vi "XNET Create Timing Source (FlexRay Cycle).vi"(0 "session in":refnum<k21>, 1 "timing source name":string, 7 "macrotick offset":u32, 11 "error in (no error)":errorcluster) -> (4 "session out":refnum<k21>, 6 "timing source out":string, 15 "error out":errorcluster)   [LabVIEW 2018]
doc: "Creates a timing source for a Timed Loop on LabVIEW Real-Time.\n\nThe timing source is based on the FlexRay communication cycle. The timing source sends a tick to the Timed Loop at a specific offset in time within the FlexRay cycle. The offset within the cycle is specified in FlexRay macroticks."
uses:
  nixlvapi.dll
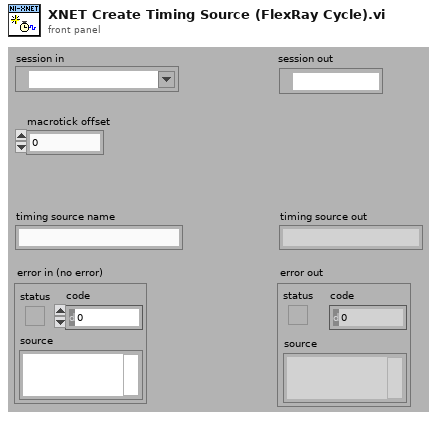
[diagram p1: front panel]
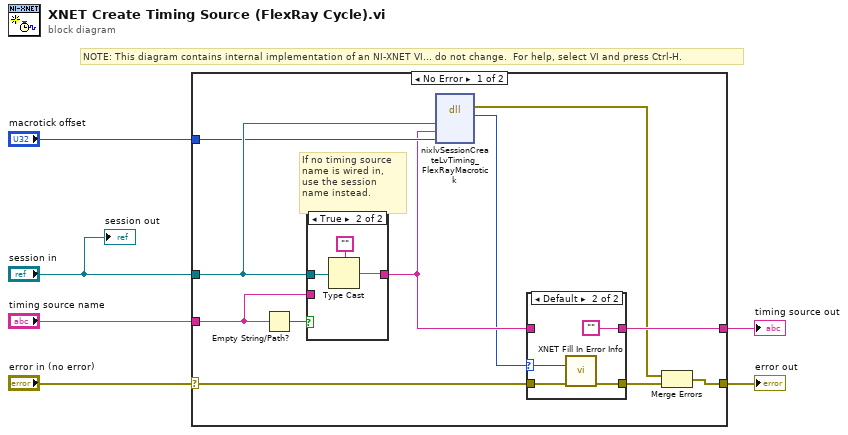
[diagram p0: block diagram]
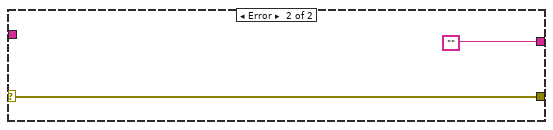
[diagram p4: hidden frame]
diagram:
  # "NOTE: This diagram contains internal implementation of an NI-XNET VI... do not change.  For help, select VI and press Ctrl-H."
  n1 = case shown="No Error" "error in (no error)" {
    selector: "error in (no error)" -> [w17 w29]
    tunnel: [w8 w29] -> w5
    tunnel: "timing source name" -> [w14 _]
    tunnel: "session in" -> [w12 _]
    tunnel: "macrotick offset" -> [w11 _]
    tunnel: [w13 ""] -> w1
    frame No Error {
      # "If no timing source \nname is wired in,\nuse the session \nname instead."
      # "NOTE: This diagram contains internal implementation of an NI-XNET VI... do not change.  For help, select VI and press Ctrl-H."
      n2 = Empty String/Path?(string/path=w14) -> (empty?=w15:bool)
      n3 = case shown="True" w15 {
        tunnel: w12 -> [_ w21]
        tunnel: w14 -> [w18 _]
        tunnel: [w18 w19] -> w10
        frame False {
        }
        frame True {
          n4 = Type Cast(type="", x=w21) -> (*(type *) &x=w19:string)
        }
      }
      n5 = dll-call lib="nixlvapi.*" fn="nixlvSessionCreateLvTiming_FlexRayMacrotick" ("nilvxaiu.dll:lvxenSessionClear")("reference"=w12, "timingSourceName"=w10, "macrotickOffset"=w11) -> (error out=w7:errorcluster, "return type"=w9:i32)  [unwired: 4 in, 3 out]
      n6 = case shown="Default" w9 {
        selector: w9 -> [_ w25]
        tunnel: w17 -> [w23 w26]
        tunnel: [w23 w27] -> w16
        tunnel: [w22 ""] -> w13
        tunnel: w10 -> [w22 _]
        frame 0 {
        }
        frame Default {
          n7 = call "XNET Fill In Error Info.vi"("status code"=w25, "error in"=w26) -> ("error out"=w27:errorcluster)  [unwired: 13 out]
        }
      }
      n8 = Merge Errors(w7, w16) -> (w8:errorcluster)
    }
    frame Error {
    }
  }
  "error out" <- w5
  "timing source out" <- w1
  "session out" <- "session in"
